vi "Graph.vi"(8 "error in (no error)":errorcluster, 10 "notifier out":refnum<notifier>, 11 "Agitator Module State Cluster":T1={"State"=enum."Idle", "Start Time"=timestamp(0 s since 1904-01-01), "Current Time"=timestamp(0 s since 1904-01-01), "Agitator Module Config"={"GUID"="", "Drop Coords"={"Horizontal"=0, "Vertical"=0}, "Process Name"="", "User name"="", "Queue Name"="", "Settings"={"Cycle Period"=500.0, "Agitator Type"="", "Setpoint (µm)"=0.0, "IKA EUROSTAR Settings"={"VISA resource name"="", "Simulated?"=FALSE}}, "Load Count"=0}, "Output Error"=FALSE, "Log Started"=FALSE, "First Iteration"=FALSE, "Data"={"Agitator rpm Value"=0.0}, "Agitator On?"=enum."Off"}) -> (0 "error out":errorcluster, 3 "Agitator Module State Cluster":T1={"State"=enum."Idle", "Start Time"=timestamp(0 s since 1904-01-01), "Current Time"=timestamp(0 s since 1904-01-01), "Agitator Module Config"={"GUID"="", "Drop Coords"={"Horizontal"=0, "Vertical"=0}, "Process Name"="", "User name"="", "Queue Name"="", "Settings"={"Cycle Period"=500.0, "Agitator Type"="", "Setpoint (µm)"=0.0, "IKA EUROSTAR Settings"={"VISA resource name"="", "Simulated?"=FALSE}}, "Load Count"=0}, "Output Error"=FALSE, "Log Started"=FALSE, "First Iteration"=FALSE, "Data"={"Agitator rpm Value"=0.0}, "Agitator On?"=enum."Off"})   [LabVIEW 2018, in "Agitator Module.lvlib" / "Agitator Module Engine.lvlib"]
uses:
  Agitator Module Engine.lvlib
  Feed Module/Controls/Agitator Module State Cluster.ctl
  Pump Module Folder/Measure Instrument/State Enum.ctl
  Feed Module/Controls/Agitator Module Config Cluster.ctl
  <vilib>/Utility/miscctls.llb/LVPoint32TypeDef.ctl
  Feed Module/Controls/Agitator Module Settings Cluster.ctl
  IKA EUROSTAR/IKA EUROSTAR Settings.ctl
  Agitator Module.lvlib
  Pump Module Folder/Measure Instrument/Pump Module Engine.lvlib
  IKA EUROSTAR/IKA EUROSTAR.lvlib
panel:
  # "Agitator Settings"
  # "Agitator Settings"
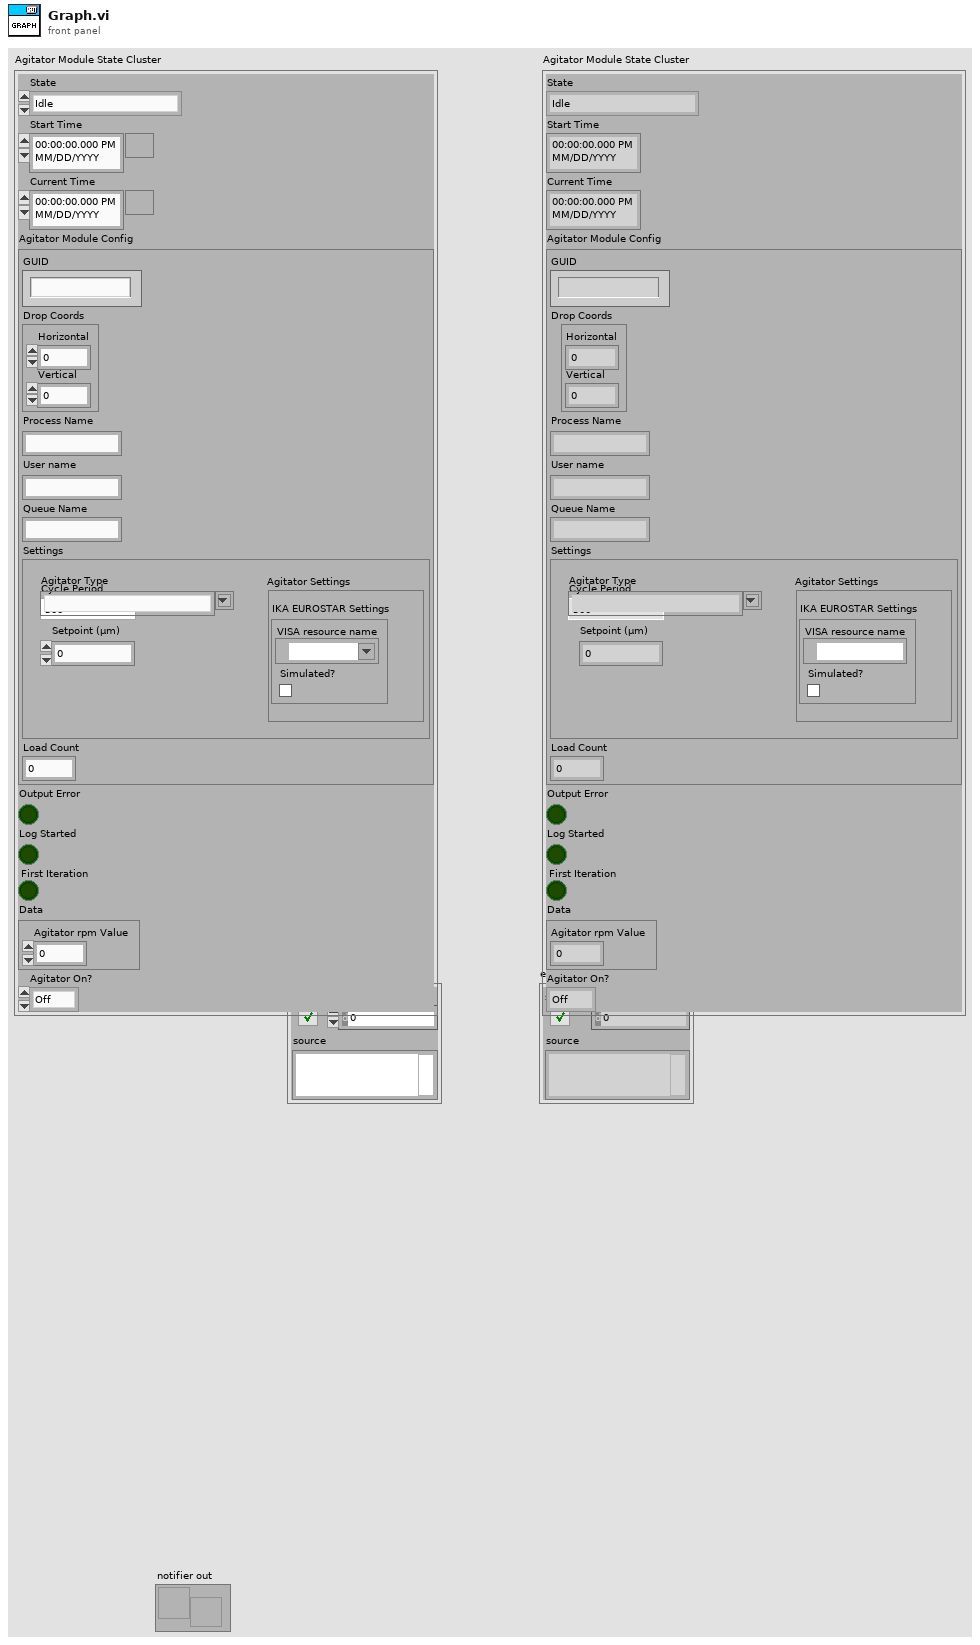
[diagram p1: front panel]
types:
  T1 = typedef "Agitator Module.lvlib/Agitator Module State Cluster.ctl" = cluster{"State":T2, "Start Time":timestamp, "Current Time":timestamp, "Agitator Module Config":T3, "Output Error":bool, "Log Started":bool, "First Iteration":bool, "Data":cluster{"Agitator rpm Value":dbl}, "Agitator On?":enum16{"Off", "On", "Not Initialized", "Over Cutoff"}}
  T2 = typedef "Pump Module.lvlib/Pump Module Engine.lvlib/State Enum.ctl" = enum16{"Measuring", "Idle", "Paused"}
  T3 = typedef "Agitator Module.lvlib/Agitator Module Config Cluster.ctl" = cluster{"GUID":string, "Drop Coords":T4, "Process Name":string, "User name":string, "Queue Name":string, "Settings":T5, "Load Count":i32}
  T4 = typedef "LVPoint32TypeDef.ctl" = cluster{"Horizontal":i32, "Vertical":i32}
  T5 = typedef "Agitator Module.lvlib/Agitator Module Settings Cluster.ctl" = cluster{"Cycle Period":dbl, "Agitator Type":string, "Setpoint (µm)":dbl, "IKA EUROSTAR Settings":T6}
  T6 = typedef "IKA EUROSTAR.lvlib/IKA EUROSTAR Settings.ctl" = cluster{"VISA resource name":refnum<visa-resource-name>, "Simulated?":bool}
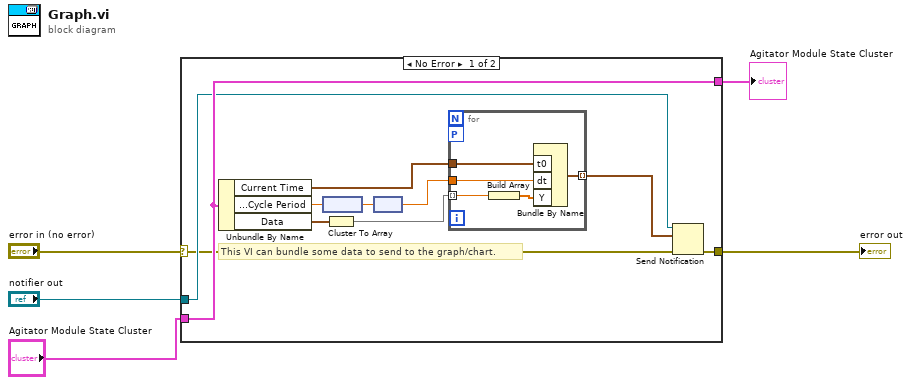
[diagram p0: block diagram]
diagram:
  n1 = case shown="No Error" "error in (no error)" {
    selector: "error in (no error)" -> [w14 w23]
    tunnel: [w13 w23] -> w4
    tunnel: "Agitator Module State Cluster" -> [w16 w22]
    tunnel: [w16 w22] -> w2
    tunnel: "notifier out" -> [w15 _]
    frame No Error {
      # "This VI can bundle some data to send to the graph/chart."
      n2 = Unbundle By Name(w16) -> ("Current Time"=w12:timestamp, "Agitator Module Config.Settings.Cycle Period"=w11:dbl, "Data"=w6:cluster{"Agitator rpm Value":dbl})
      n3 = node(w11) -> (w10:dbl[unit])
      n4 = Cluster To Array(cluster=w6) -> (array=w8:dbl[])
      n5 = node(w10) -> (w9:dbl)
      n6 = for {
        tunnel: w12 -> [w21]
        tunnel: w9 -> [w20]
        tunnel: w8 -> [w19] mode=indexing
        tunnel: [w17] -> w7 mode=indexing
        workers-P: _ -> [_]
        n7 = Build Array(w19) -> (w18:dbl[])
        n8 = Bundle By Name("t0"=w21, "dt"=w20, "Y"=w18) -> (w17:waveform(dbl))  [unwired: 1 in]
      }
      n9 = Send Notification(notification=w7, notifier=w15, error in (no error)=w14) -> (error out=w13:errorcluster)  [unwired: 1 out]
    }
    frame Error {
    }
  }
  "error out" <- w4
  "Agitator Module State Cluster" <- w2
